vi "Dpc Put Spi.vi"(0 "hif":u32, 1 "perc":i32, 5 "cbSnd":i32, 7 "rgbSnd":string, 9 "rgbRcv":string, 11 "error in (no error)":errorcluster, 12 "ptrid":u16) -> (3 "perc out":i32, 4 "hif out":u32, 6 "function return":i32, 8 "rgbSnd out":string, 10 "rgbRcv out":string, 14 "ptrid out":u16, 15 "error out":errorcluster)   [LabVIEW 2011, in "LVH-Adept.lvlib" / "DPCUTIL.lvlib"]
doc: "DPCAPI BOOL DpcPutSpi(HANDLE hif, INT32 cbSnd, BYTE * rgbSnd, BYTE * rgbRcv, ERC * perc, TRID * ptrid);"
uses:
  DPCUTIL.lvlib
  dpcutil.dll
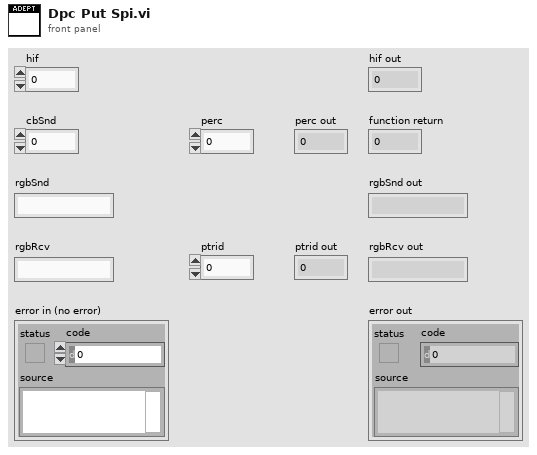
[diagram p1: front panel]
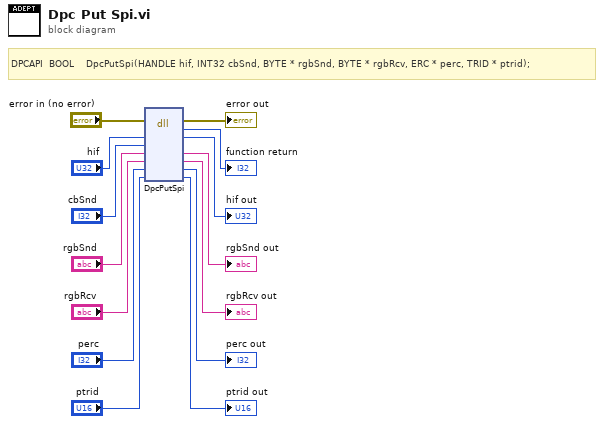
[diagram p0: block diagram]
diagram:
  # "DPCAPI  BOOL    DpcPutSpi(HANDLE hif, INT32 cbSnd, BYTE * rgbSnd, BYTE * rgbRcv, ERC * perc, TRID * ptrid);"
  n1 = dll-call lib="dpcutil.*" fn="DpcPutSpi"(error in="error in (no error)", "hif"="hif", "cbSnd"="cbSnd", "rgbSnd"="rgbSnd", "rgbRcv"="rgbRcv", "perc"="perc", "ptrid"="ptrid") -> (error out=→"error out":errorcluster, →"function return":i32, "hif"=→"hif out":u32, "rgbSnd"=→"rgbSnd out":string, "rgbRcv"=→"rgbRcv out":string, "perc"=→"perc out":i32, "ptrid"=→"ptrid out":u16)  [unwired: 3 in, 1 out]
